vi "Set Output Format.vi"(8 "error in (no error)":errorcluster, 9 "alignment (none)":enum16{"None", "Left", "Center", "Right"}(ring), 10 "auto wrap? (F)":bool, 11 "LCD in":refnum<class "Character LCD.lvclass">) -> (0 "error out":errorcluster, 3 "LCD out":refnum<class "Character LCD.lvclass">)   [LabVIEW 2015, in "HD44780 Host.lvlib"]
uses:
  HD44780 Host.lvlib
  Internal/LCD Class/Character LCD.lvclass
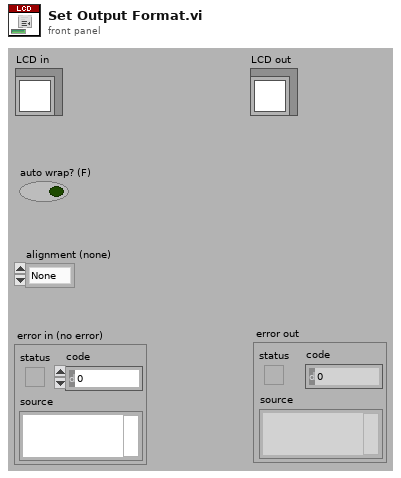
[diagram p1: front panel]
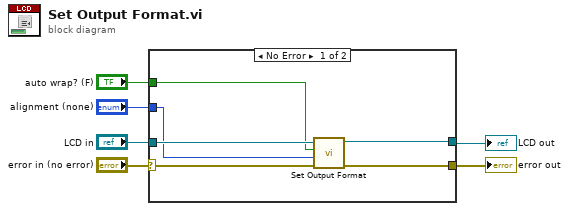
[diagram p0: block diagram]
diagram:
  n1 = case shown="No Error" "error in (no error)" {
    selector: "error in (no error)" -> [w12 w13]
    tunnel: [w10 w13] -> w5
    tunnel: "LCD in" -> [w11 w14]
    tunnel: [w9 w14] -> w3
    tunnel: "alignment (none)" -> [w8 _]
    tunnel: "auto wrap? (F)" -> [w7 _]
    frame No Error {
      n2 = call-dynamic "Set Output Format.vi"("error in (no error)"=w12, "alignment (none)"=w8, "auto wrap? (F)"=w7, "Character LCD in"=w11) -> ("error out"=w10:errorcluster, "Character LCD out"=w9:refnum<class "Character LCD.lvclass">)  [unwired: 6 in]
    }
    frame Error {
    }
  }
  "error out" <- w5
  "LCD out" <- w3
